vi "Set Parameter.vi"(4 "RingText.Text":string, 6 "txtpower":dbl, 7 "txtstepwave":dbl, 8 "error in":errorcluster, 9 "txtstopwave":dbl, 10 "txtstartwave":dbl, 11 "Address Cluster":T1 {"tsl_communcation_method" items=["GPIB", "C232C", "TCPIP", "USB"]; "MPM_communcation_method" items=["GPIB", "C232C", "TCPIP", "USB"]}) -> (0 "error out":errorcluster, 3 "ILSTS":refnum<k24>)   [LabVIEW 2017]
uses:
  CTL/Address Cluster.ctl
  D:/test/ILSTS/LV_IL_Sample/DLL/InstrumentDLL.dll
  DLL/InstrumentDLL.dll
  D:/test/ILSTS/LV_IL_Sample/DLL/STSProcess.dll
  DLL/STSProcess.dll
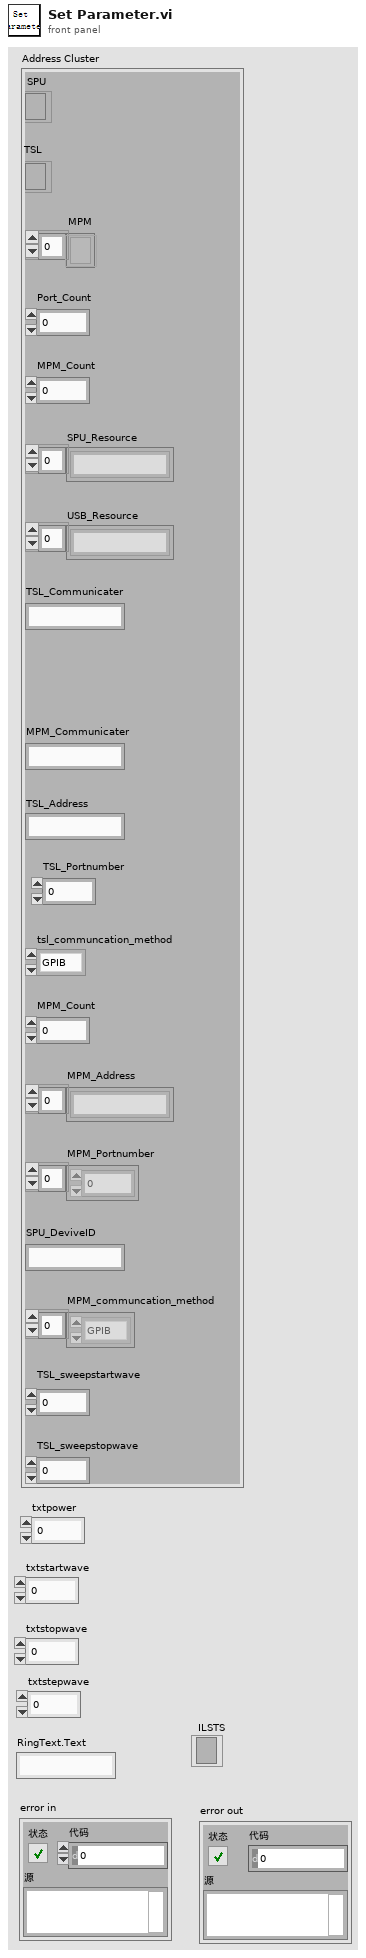
[diagram p1: front panel]
types:
  T1 = typedef "Address Cluster.ctl" = cluster{"SPU":refnum<k24>, "MPM":refnum<k24>[], "Port_Count":dbl, "MPM_Count":dbl, "SPU_Resource":string[], "USB_Resource":string[], "MPM_Communicater":string, "MPM_Count":dbl, "MPM_Address":string[], "MPM_Portnumber":dbl[], "SPU_DeviveID":string, "MPM_communcation_method":i32[], "TSL_sweepstartwave":dbl, "TSL_sweepstopwave":dbl, "TSL_Address":string, "TSL_Communicater":string, "TSL":refnum<k24>, "tsl_communcation_method":i32, "TSL_Portnumber":dbl}
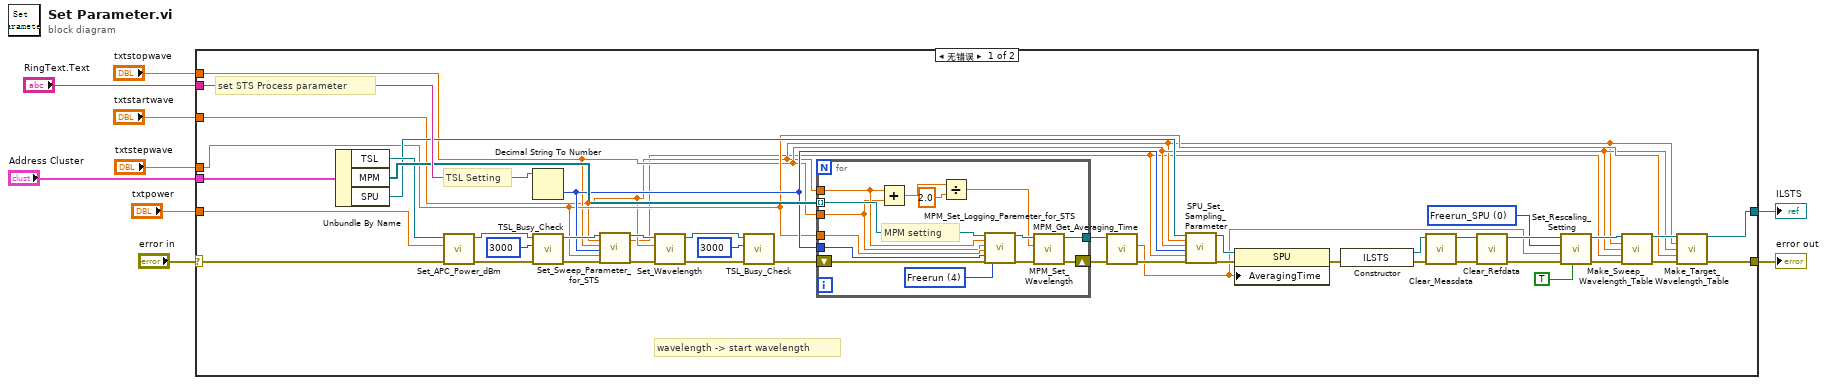
[diagram p0: block diagram]
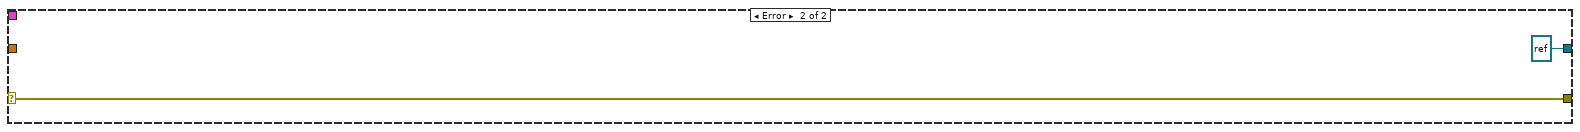
[diagram p2: hidden frame]
diagram:
  n1 = case shown="无错误" "error in" {
    selector: "error in" -> [w49 w69]
    tunnel: "txtstepwave" -> [w19 _]
    tunnel: "RingText.Text" -> [w53 _]
    tunnel: "txtpower" -> [w52 _]
    tunnel: [w16 refnum<k24> refnum ("STSProcess.ILSTS")] -> w1
    tunnel: "Address Cluster" -> [w50 _]
    tunnel: [w48 w69] -> w4
    tunnel: "txtstopwave" -> [w18 _]
    tunnel: "txtstartwave" -> [w17 _]
    frame No Error {
      w35 = 0 items=["Freerun_SPU", "Freerun_Referencemodule"] ("mode")
      # "set STS Process parameter"
      # "wavelength -> start wavelength"
      # "TSL Setting"
      n2 = Unbundle By Name(w50) -> ("TSL"=w28:refnum<k24>, "MPM"=w51:refnum<k24>[], "SPU"=w24:refnum<k24>)
      n3 = call "Set_APC_Power_dBm.vi"(".NET Reference in"=w28, "Setting Power"=w52, "error in (no error)"=w49) -> ("Reference out"=w46:refnum<k24>, "error out"=w47:errorcluster)  [unwired: 6 in]
      n4 = Decimal String To Number(string=w53) -> (number=w22:i32)  [unwired: 2 in, 1 out]
      n5 = call "TSL_Busy_Check.vi"("error in (no error)"=w47, "Wait time(msec)"=3000, ".NET Reference in"=w46) -> ("error out"=w44:errorcluster, "Reference out"=w43:refnum<k24>)  [unwired: 7 in]
      n6 = call "Set_Sweep_Parameter_for_STS.vi"(".NET Reference in"=w43, "startwave"=w17, "stopwave"=w18, "speed"=w22, "rescalingstep"=w19, "error in (no error)"=w44) -> ("Reference out"=w42:refnum<k24>, "acctualstep"=w10:dbl, "error out"=w41:errorcluster)  [unwired: 11 in]
      n7 = call "Set_Wavelength.vi"("error in (no error)"=w41, "txtsetwave"=w17, ".NET Reference in"=w42) -> ("error out"=w27:errorcluster, "Reference out"=w20:refnum<k24>)  [unwired: 3 in]
      n8 = call "TSL_Busy_Check.vi"("error in (no error)"=w27, "Wait time(msec)"=3000, ".NET Reference in"=w20) -> ("error out"=w26:errorcluster)  [unwired: 7 in, 1 out]
      n9 = for {
        tunnel: w51 -> [w67] mode=indexing
        tunnel: w17 -> [w58]
        tunnel: w18 -> [w57]
        tunnel: w22 -> [w65]
        tunnel: w19 -> [w63]
        shift-right: [w61] -> w29
        shift-left: w26 -> [w66]
        tunnel: [w60] -> w30
        w64 = 4 items=["ManualRangeConstant", "ManualRangeSweep", "AutoRangeConstant", "AutoRangeSweep", "Freerun"] ("mode")
        # "MPM setting"
        n10 = Add(x=w58, y=w57) -> (x+y=w56:dbl)
        n11 = Divide(x=w56, y=2.0) -> (x/y=w54:dbl)
        n12 = call "MPM_Set_Logging_Paremeter_for_STS.vi"(".NET Reference in"=w67, "startwave"=w58, "stopwave"=w57, "wavestep"=w63, "speed"=w65, "error in (no error)"=w66, "mode"=w64) -> ("Reference out"=w59:refnum<k24>, "error out"=w62:errorcluster)  [unwired: 11 in]
        n13 = call "MPM_Set_Wavelength.vi"("error in (no error)"=w62, "Wavelength(nm)"=w54, ".NET Reference in"=w59) -> ("error out"=w61:errorcluster, "Reference out"=w60:refnum<k24>)  [unwired: 7 in]
      }
      n14 = call "MPM_Get_Averaging_Time.vi"("error in (no error)"=w29, ".NET Reference in"=w30) -> ("error out"=w23:errorcluster, "time out"=w11:dbl)  [unwired: 7 in, 1 out]
      n15 = call "SPU_Set_Sampling_Parameter.vi"("引用"=w24, "startwave"=w17, "stopwave"=w18, "speed"=w22, "triggerstep"=w10, "错误输入（无错误）"=w23) -> ("引用输出"=w12:refnum<k24>, "error IO"=w15:errorcluster)  [unwired: 12 in]
      n16 = property class="SPU"(reference=w12, error in=w15, "AveragingTime"=w11) -> (error out=w14:errorcluster)  [unwired: 1 out]
      n17 = constructor class="ILSTS"(error in=w14) -> (reference out=w21:refnum<k24>, error out=w13:errorcluster)  [unwired: 2 in, 1 out]
      n18 = call "Clear_Measdata.vi"("error in (no error)"=w13, ".NET Reference in"=w21) -> ("error out"=w39:errorcluster, "Reference out"=w40:refnum<k24>)  [unwired: 8 in]
      n19 = call "Clear_Refdata.vi"("error in (no error)"=w39, ".NET Reference in"=w40) -> ("error out"=w37:errorcluster, "Reference out"=w38:refnum<k24>)  [unwired: 8 in]
      n20 = call "Set_Rescaling_Setting.vi"("isOriginalMonitor"=TRUE, "error in (no error)"=w37, "avg"=w11, "mode"=w35, ".NET Reference in"=w38) -> ("error out"=w33:errorcluster, "Reference out"=w34:refnum<k24>)  [unwired: 5 in]
      n21 = call "Make_Sweep_Wavelength_Table.vi"(".NET Reference in"=w34, "startwave"=w17, "endwave"=w18, "triggerstep"=w10, "error in (no error)"=w33) -> ("Reference out"=w32:refnum<k24>, "error out"=w31:errorcluster)  [unwired: 9 in]
      n22 = call "Make_Target_Wavelength_Table.vi"(".NET Reference in"=w32, "startwave"=w17, "endwave"=w18, "targetdatastep"=w19, "error in (no error)"=w31) -> ("Reference out"=w16:refnum<k24>, "error out"=w48:errorcluster)  [unwired: 9 in]
    }
    frame Error {
    }
  }
  "error out" <- w4
  "ILSTS" <- w1
